vi "ExSubSetCalibInSpeFileHeader.vi"(3 "error in (no error)":errorcluster, 4 "Calibration Handle":u32, 5 "File Handle":u32) -> (0 "error out":errorcluster, 1 "Calibration Handle":u32, 2 "File Handle":u32)   [LabVIEW 2010]
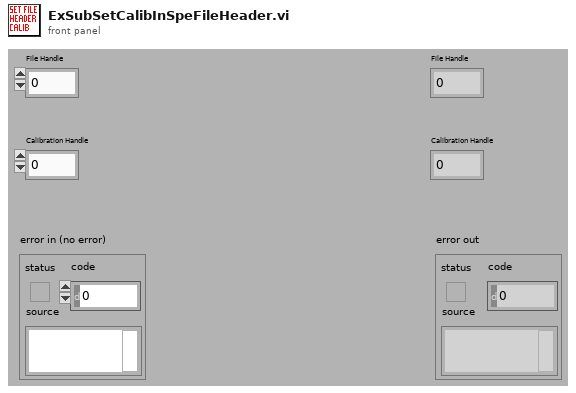
[diagram p1: front panel]
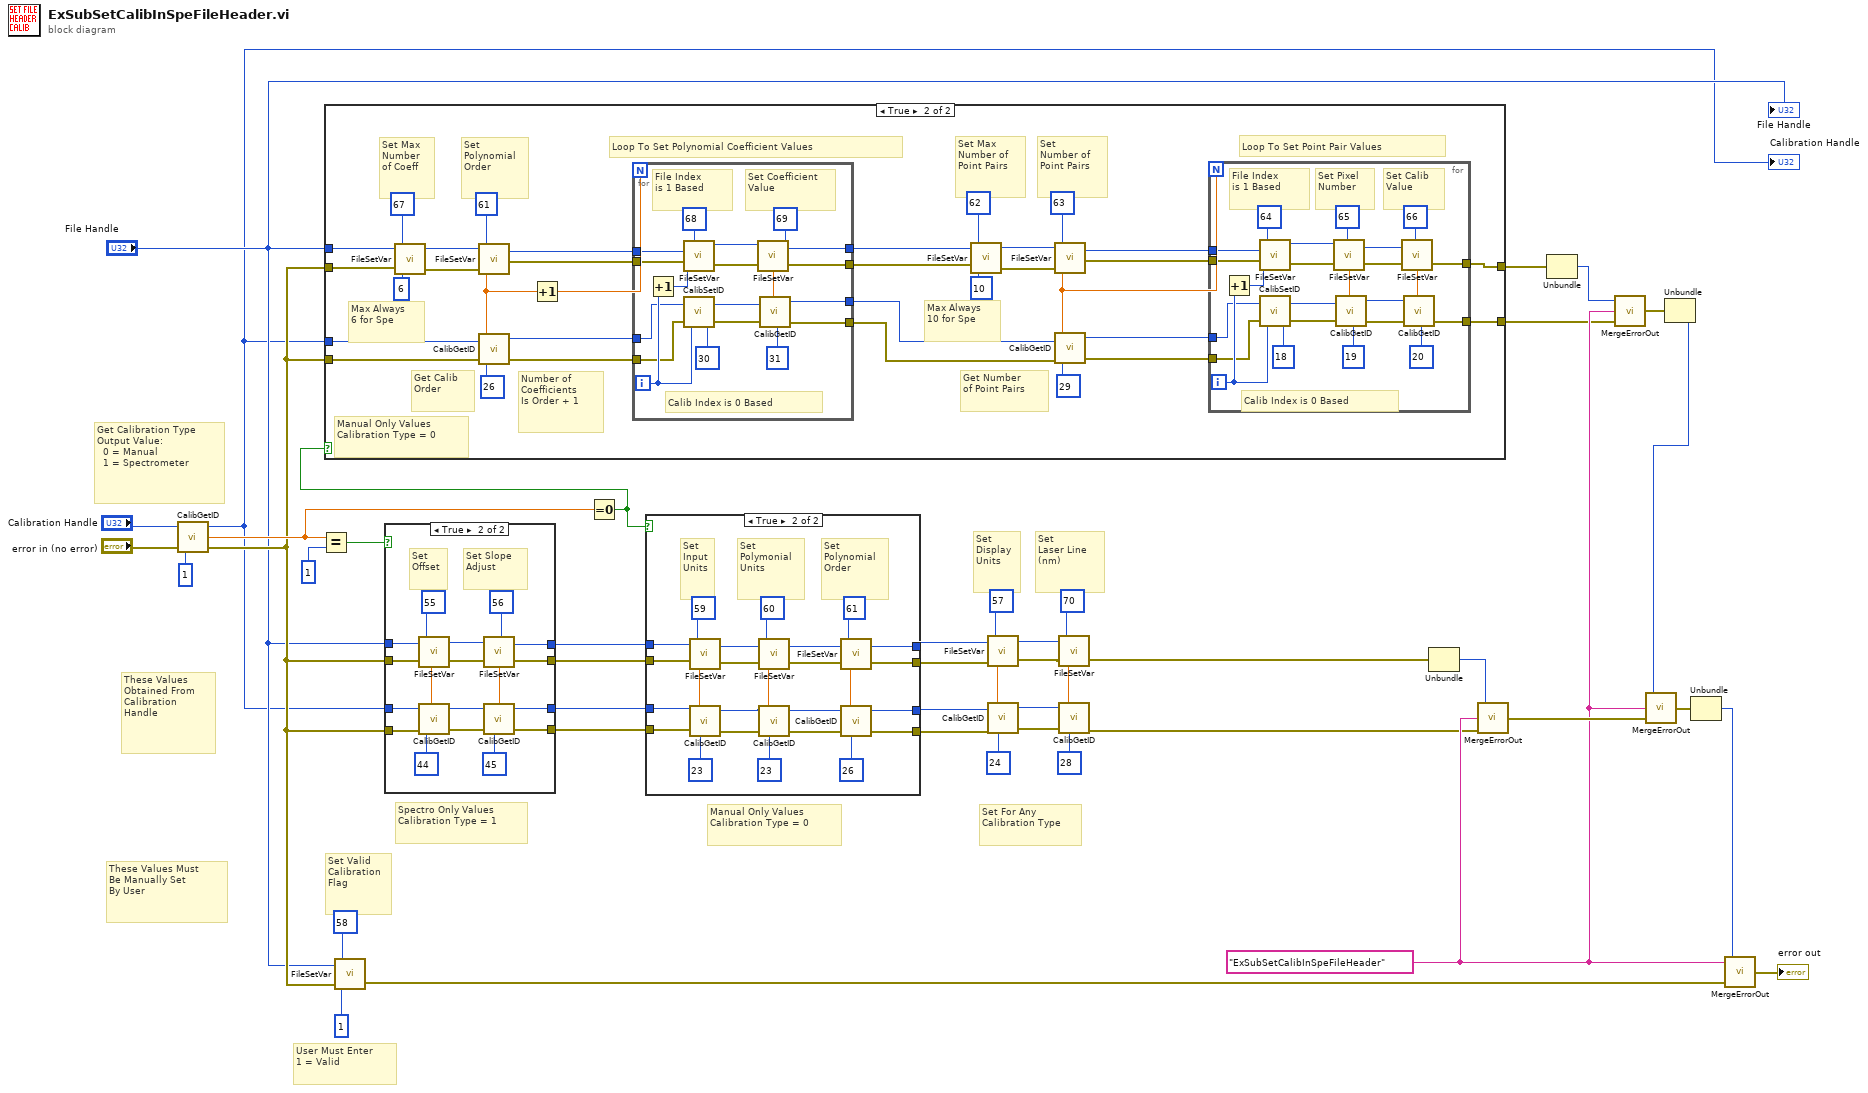
[diagram p0: block diagram]
diagram:
  w27 = "ExSubSetCalibInSpeFileHeader"
  # "Set For Any\nCalibration Type"
  # "Manual Only Values\nCalibration Type = 0"
  # "Spectro Only Values\nCalibration Type = 1"
  # "Get Calibration Type\nOutput Value:\n  0 = Manual\n  1 = Spectrometer"
  # "These Values Must\nBe Manually Set\nBy User"
  # "These Values\nObtained From\nCalibration\nHandle"
  # "User Must Enter\n1 = Valid"
  # "Set Valid\nCalibration\nFlag"
  # "Set\nLaser Line\n(nm)"
  # "Set\nDisplay\nUnits"
  n1 = call <userlib>:"CalibGetID.vi"("error in"="error in (no error)", "Enumerated ID"=1, "Calibration Handle"="Calibration Handle") -> ("error out"=w8:errorcluster, "Value From Calibration"=w21:dbl, "Calibration Handle"=w6:u32)
  "Calibration Handle" <- w6
  n2 = Equal?(x=w21, y=1) -> (x = y?=w22:bool)
  n3 = call <userlib>:"FileSetVar.vi"("error in"=w8, "Value"=1, "Parameter ID"=58, "File Handle"="File Handle") -> ("error out"=w31:errorcluster)  [unwired: 1 out]
  n4 = case shown="True" w22 {
    tunnel: w6 -> [w45 w58]
    tunnel: [w45 w57] -> w18
    tunnel: w8 -> [w46 w56]
    tunnel: [w46 w55] -> w17
    tunnel: "File Handle" -> [w48 w52]
    tunnel: [w48 w51] -> w20
    tunnel: w8 -> [w47 w50]
    tunnel: [w47 w49] -> w19
    frame False {
    }
    frame True {
      # "Set Slope\nAdjust"
      # "Set\nOffset"
      n5 = call <userlib>:"CalibGetID.vi"("error in"=w56, "Enumerated ID"=44, "Calibration Handle"=w58) -> ("error out"=w60:errorcluster, "Value From Calibration"=w64:dbl, "Calibration Handle"=w61:u32)
      n6 = call <userlib>:"FileSetVar.vi"("error in"=w50, "Value"=w64, "Parameter ID"=55, "File Handle"=w52) -> ("error out"=w59:errorcluster, "File Handle"=w63:u32)
      n7 = call <userlib>:"CalibGetID.vi"("error in"=w60, "Enumerated ID"=45, "Calibration Handle"=w61) -> ("error out"=w55:errorcluster, "Value From Calibration"=w54:dbl, "Calibration Handle"=w57:u32)
      n8 = call <userlib>:"FileSetVar.vi"("error in"=w59, "Value"=w54, "Parameter ID"=56, "File Handle"=w63) -> ("error out"=w49:errorcluster, "File Handle"=w51:u32)
    }
  }
  n9 = Equal To 0?(x=w21) -> (x = 0?=w3:bool)
  n10 = case shown="True" w3 {
    tunnel: w8 -> [w68 w74]
    tunnel: w8 -> [w67 w73]
    tunnel: "File Handle" -> [_ w72]
    tunnel: w6 -> [_ w71]
    tunnel: [w67 w70] -> w5
    tunnel: [w68 w69] -> w4
    frame False {
    }
    frame True {
      # "Manual Only Values\nCalibration Type = 0"
      # "Max Always\n10 for Spe"
      # "Get Number\nof Point Pairs"
      # "Loop To Set Point Pair Values"
      # "Set\nNumber of\nPoint Pairs"
      # "Set Max\nNumber of\nPoint Pairs"
      # "Max Always\n6 for Spe"
      # "Get Calib\nOrder"
      # "Loop To Set Polynomial Coefficient Values"
      # "Number of\nCoefficients\nIs Order + 1"
      # "Set\nPolynomial\nOrder"
      # "Set Max\nNumber\nof Coeff"
      n11 = call <userlib>:"FileSetVar.vi"("error in"=w74, "Value"=6, "Parameter ID"=67, "File Handle"=w72) -> ("error out"=w96:errorcluster, "File Handle"=w97:u32)
      n12 = call <userlib>:"CalibGetID.vi"("error in"=w73, "Enumerated ID"=26, "Calibration Handle"=w71) -> ("error out"=w90:errorcluster, "Value From Calibration"=w95:dbl, "Calibration Handle"=w91:u32)
      n13 = call <userlib>:"FileSetVar.vi"("error in"=w96, "Value"=w95, "Parameter ID"=61, "File Handle"=w97) -> ("error out"=w92:errorcluster, "File Handle"=w93:u32)
      n14 = Increment(x=w95) -> (x+1=w94:dbl)
      n15 = for {
        N: w94 -> [_]
        tunnel: w93 -> [w132]
        tunnel: w92 -> [w131]
        tunnel: w91 -> [w140]
        tunnel: w90 -> [w142]
        tunnel: [w130] -> w79
        tunnel: [w129] -> w75
        tunnel: [w128] -> w77
        tunnel: [w127] -> w78
        i -> [w144]
        # "Set Coefficient\nValue"
        # "Calib Index is 0 Based"
        # "File Index\nis 1 Based"
        n16 = Increment(x=w144) -> (x+1=w143:i32)
        n17 = call <userlib>:"FileSetVar.vi"("error in"=w131, "Value"=w143, "Parameter ID"=68, "File Handle"=w132) -> ("error out"=w134:errorcluster, "File Handle"=w133:u32)
        n18 = call <userlib>:"CalibSetID.vi"("error in"=w142, "Value To Set"=w144, "Enumerated ID"=30, "Calibration Handle"=w140) -> ("error out"=w141:errorcluster, "Calibration Handle"=w139:u32)
        n19 = call <userlib>:"CalibGetID.vi"("error in"=w141, "Enumerated ID"=31, "Calibration Handle"=w139) -> ("error out"=w127:errorcluster, "Value From Calibration"=w135:dbl, "Calibration Handle"=w128:u32)
        n20 = call <userlib>:"FileSetVar.vi"("error in"=w134, "Value"=w135, "Parameter ID"=69, "File Handle"=w133) -> ("error out"=w129:errorcluster, "File Handle"=w130:u32)
      }
      n21 = call <userlib>:"FileSetVar.vi"("error in"=w75, "Value"=10, "Parameter ID"=62, "File Handle"=w79) -> ("error out"=w85:errorcluster, "File Handle"=w86:u32)
      n22 = call <userlib>:"CalibGetID.vi"("error in"=w78, "Enumerated ID"=29, "Calibration Handle"=w77) -> ("error out"=w81:errorcluster, "Value From Calibration"=w80:dbl, "Calibration Handle"=w82:u32)
      n23 = call <userlib>:"FileSetVar.vi"("error in"=w85, "Value"=w80, "Parameter ID"=63, "File Handle"=w86) -> ("error out"=w83:errorcluster, "File Handle"=w84:u32)
      n24 = for {
        N: w80 -> [_]
        tunnel: w84 -> [w113]
        tunnel: w83 -> [w112]
        tunnel: w82 -> [w121]
        tunnel: w81 -> [w123]
        tunnel: [w103] -> w69
        tunnel: [w102] -> w70
        i -> [w125]
        # "Set Calib\nValue"
        # "Set Pixel\nNumber"
        # "Calib Index is 0 Based"
        # "File Index\nis 1 Based"
        n25 = Increment(x=w125) -> (x+1=w124:i32)
        n26 = call <userlib>:"FileSetVar.vi"("error in"=w112, "Value"=w124, "Parameter ID"=64, "File Handle"=w113) -> ("error out"=w115:errorcluster, "File Handle"=w114:u32)
        n27 = call <userlib>:"CalibSetID.vi"("error in"=w123, "Value To Set"=w125, "Enumerated ID"=18, "Calibration Handle"=w121) -> ("error out"=w122:errorcluster, "Calibration Handle"=w120:u32)
        n28 = call <userlib>:"CalibGetID.vi"("error in"=w122, "Enumerated ID"=19, "Calibration Handle"=w120) -> ("error out"=w104:errorcluster, "Value From Calibration"=w116:dbl, "Calibration Handle"=w105:u32)
        n29 = call <userlib>:"FileSetVar.vi"("error in"=w115, "Value"=w116, "Parameter ID"=65, "File Handle"=w114) -> ("error out"=w106:errorcluster, "File Handle"=w107:u32)
        n30 = call <userlib>:"CalibGetID.vi"("error in"=w104, "Enumerated ID"=20, "Calibration Handle"=w105) -> ("error out"=w102:errorcluster, "Value From Calibration"=w108:dbl)  [unwired: 1 out]
        n31 = call <userlib>:"FileSetVar.vi"("error in"=w106, "Value"=w108, "Parameter ID"=66, "File Handle"=w107) -> ("error out"=w103:errorcluster)  [unwired: 1 out]
      }
    }
  }
  n32 = case shown="True" w3 {
    tunnel: w20 -> [w148 w153]
    tunnel: w19 -> [w147 w154]
    tunnel: w18 -> [w146 w155]
    tunnel: w17 -> [w145 w156]
    tunnel: [w148 w152] -> w16
    tunnel: [w147 w151] -> w15
    tunnel: [w146 w150] -> w14
    tunnel: [w145 w149] -> w13
    frame False {
    }
    frame True {
      # "Set\nPolynomial\nOrder"
      # "Set\nPolymonial\nUnits"
      # "Set\nInput\nUnits"
      n33 = call <userlib>:"CalibGetID.vi"("error in"=w156, "Enumerated ID"=23, "Calibration Handle"=w155) -> ("error out"=w158:errorcluster, "Value From Calibration"=w171:dbl, "Calibration Handle"=w160:u32)
      n34 = call <userlib>:"FileSetVar.vi"("error in"=w154, "Value"=w171, "Parameter ID"=59, "File Handle"=w153) -> ("error out"=w162:errorcluster, "File Handle"=w164:u32)
      n35 = call <userlib>:"CalibGetID.vi"("error in"=w158, "Enumerated ID"=23, "Calibration Handle"=w160) -> ("error out"=w157:errorcluster, "Value From Calibration"=w168:dbl, "Calibration Handle"=w159:u32)
      n36 = call <userlib>:"FileSetVar.vi"("error in"=w162, "Value"=w168, "Parameter ID"=60, "File Handle"=w164) -> ("error out"=w161:errorcluster, "File Handle"=w163:u32)
      n37 = call <userlib>:"CalibGetID.vi"("error in"=w157, "Enumerated ID"=26, "Calibration Handle"=w159) -> ("error out"=w149:errorcluster, "Value From Calibration"=w165:dbl, "Calibration Handle"=w150:u32)
      n38 = call <userlib>:"FileSetVar.vi"("error in"=w161, "Value"=w165, "Parameter ID"=61, "File Handle"=w163) -> ("error out"=w151:errorcluster, "File Handle"=w152:u32)
    }
  }
  n39 = call <userlib>:"CalibGetID.vi"("error in"=w13, "Enumerated ID"=24, "Calibration Handle"=w14) -> ("error out"=w12:errorcluster, "Value From Calibration"=w42:dbl, "Calibration Handle"=w11:u32)
  n40 = call <userlib>:"FileSetVar.vi"("error in"=w15, "Value"=w42, "Parameter ID"=57, "File Handle"=w16) -> ("error out"=w10:errorcluster, "File Handle"=w9:u32)
  n41 = call <userlib>:"CalibGetID.vi"("error in"=w12, "Enumerated ID"=28, "Calibration Handle"=w11) -> ("error out"=w1:errorcluster, "Value From Calibration"=w39:dbl)  [unwired: 1 out]
  n42 = call <userlib>:"FileSetVar.vi"("error in"=w10, "Value"=w39, "Parameter ID"=70, "File Handle"=w9) -> ("error out"=w2:errorcluster)  [unwired: 1 out]
  n43 = Unbundle(w2) -> ("code"=w36:i32)  [unwired: 2 out]
  n44 = call <userlib>:"MergeErrorOut.vi"("error in"=w1, "Fucntion Name"=w27, "ErrorCode"=w36) -> ("error out"=w34:errorcluster)
  n45 = Unbundle(w4) -> ("code"=w30:i32)  [unwired: 2 out]
  n46 = call <userlib>:"MergeErrorOut.vi"("error in"=w5, "Fucntion Name"=w27, "ErrorCode"=w30) -> ("error out"=w29:errorcluster)
  n47 = Unbundle(w29) -> ("code"=w28:i32)  [unwired: 2 out]
  n48 = call <userlib>:"MergeErrorOut.vi"("error in"=w34, "Fucntion Name"=w27, "ErrorCode"=w28) -> ("error out"=w33:errorcluster)
  n49 = Unbundle(w33) -> ("code"=w32:i32)  [unwired: 2 out]
  n50 = call <userlib>:"MergeErrorOut.vi"("error in"=w31, "Fucntion Name"=w27, "ErrorCode"=w32) -> ("error out"=→"error out":errorcluster)
  "File Handle" <- "File Handle"
